vi "Logger Test.vi"   [LabVIEW 2014]
uses:
  Core/LabVIEW CI Service/Classes/Log File/Log File.lvclass
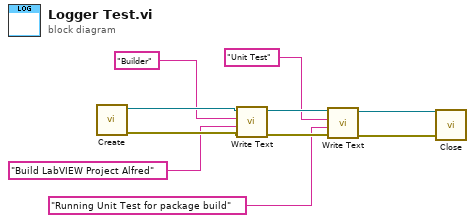
[diagram p0: block diagram]
diagram:
  n1 = call "Create.vi"() -> ("error out"=w10:errorcluster, "Log File Ref"=w9:refnum<data-value>)  [unwired: 10 in]
  n2 = call "Write Text.vi"("error in (no error)"=w10, "Text"="Build LabVIEW Project Alfred", "Header"="Builder", "Log File Ref"=w9) -> ("error out"=w5:errorcluster, "Log File Ref"=w6:refnum<data-value>)  [unwired: 6 in]
  n3 = call "Write Text.vi"("error in (no error)"=w5, "Text"="Running Unit Test for package build", "Header"="Unit Test", "Log File Ref"=w6) -> ("error out"=w3:errorcluster, "Log File Ref"=w4:refnum<data-value>)  [unwired: 6 in]
  n4 = call "Close.vi"("error in (no error)"=w3, "Log File Ref"=w4) -> ()  [unwired: 9 in, 1 out]
